vi "CreateProjectsForEachLibrary.vi"() -> ()   [LabVIEW 2023, in "Reusables.lvlib"]
uses:
  Reusables/Reusables.lvlib
  <userlib>/_OpenG.lib/file/file.llb/File Exists - Scalar__ogtk.vi
  <userlib>/_OpenG.lib/file/file.llb/openg_file.lvlib
panel:
  out "error out":errorcluster
  in  "Build Specs Folder Path":path=path "E:/sw-deps-monitor/Source/BuildSpecs"
  in  "error in (no error)":errorcluster
  in  "Source Folder Path":path=path "E:/sw-deps-monitor/Source"
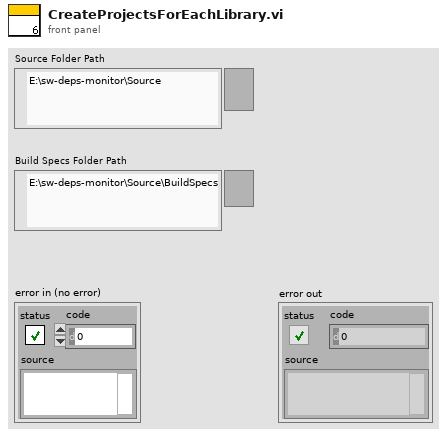
[diagram p1: front panel]
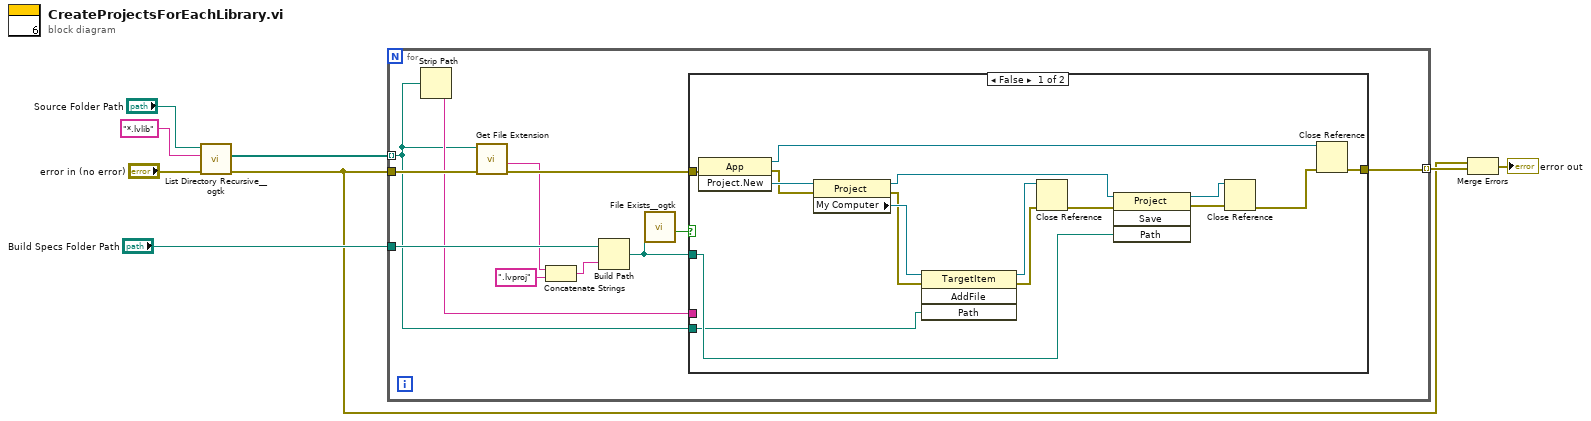
[diagram p0: block diagram]
diagram:
  n1 = call <userlib>:"List Directory Recursive__ogtk.vi"("error in (no error)"="error in (no error)", "pattern"="*.lvlib", "Path"="Source Folder Path") -> ("error out"=w2:errorcluster, "file paths"=w5:path[])  [unwired: 5 in, 2 out]
  n2 = for {
    tunnel: w2 -> [w19]
    tunnel: w5 -> [w9] mode=indexing
    tunnel: "Build Specs Folder Path" -> [w17]
    tunnel: [w12] -> w3 mode=indexing
    n3 = Strip Path(path=w9) -> (name=w13:string)  [unwired: 1 out]
    n4 = call <vilib>:"Get File Extension.vi"("error in (no error)"=w19, "file"=w9) -> ("error out"=w18:errorcluster, "filename without extension"=w16:string)  [unwired: 5 in, 3 out]
    n5 = Concatenate Strings(w16, ".lvproj" ("string")) -> (w14:string)
    n6 = Build Path(base path=w17, name or relative path=w14) -> (appended path=w11:path)
    n7 = call-poly <userlib>:"File Exists__ogtk.vi"("file path"=w11) -> ("exists"=w10:bool)  [unwired: 6 in, 1 out]
    n8 = case shown="False" w10 {
      tunnel: w18 -> [w31 w36]
      tunnel: w13 -> [_ _]
      tunnel: w9 -> [w20 _]
      tunnel: [w26 w36] -> w12
      tunnel: w11 -> [w21 _]
      frame False {
        n9 = invoke class="App" method="Project.New"(error in=w31) -> (reference out=w34:refnum<vi>, error out=w33:errorcluster, "Project:New"=w35:refnum<vi>)  [unwired: 2 in]
        n10 = property class="Project"(reference=w35, error in=w33) -> (reference out=w24:refnum<vi>, error out=w30:errorcluster, "My Computer"=w32:refnum<vi>)
        n11 = invoke class="TargetItem" method="AddFile"(reference=w32, error in=w30, "Path"=w20) -> (reference out=w29:refnum<vi>, error out=w28:errorcluster)  [unwired: 1 in, 2 out]
        n12 = Close Reference(reference=w29, error in (no error)=w28) -> (error out=w25:errorcluster)
        n13 = invoke class="Project" method="Save"(reference=w24, error in=w25, "Path"=w21) -> (reference out=w23:refnum<vi>, error out=w22:errorcluster)  [unwired: 1 in, 2 out]
        n14 = Close Reference(reference=w23, error in (no error)=w22) -> (error out=w27:errorcluster)
        n15 = Close Reference(reference=w34, error in (no error)=w27) -> (error out=w26:errorcluster)
      }
      frame True {
      }
    }
  }
  n16 = Merge Errors(w2, w3) -> (→"error out":errorcluster)
